vi "Read_HGB2.vi"(8 "error in (no error)":errorcluster, 11 "Task Array":refnum<k21>[](array[refnum])=["", ""]) -> (0 "error out":errorcluster={"status"=TRUE, "code"=-200478, "source"="Read_HGB.vi<append>\n<B>Task Name: </B>_unnamedTask<37>"}, 1 "NI 6001":waveform(dbl)[](array[waveform]), 3 "Data Main":waveform(dbl)[](array[waveform]))   [LabVIEW 2016]
uses:
  <vilib>/Utility/error.llb/DialogType.ctl
  <vilib>/DAQmx/read.llb/DAQmx Read (Analog 1D Wfm NChan NSamp).vi
  <vilib>/DAQmx/miscellaneous.llb/DAQmx Fill In Error Info.vi
panel:
  out "Accelerometer Data":waveform(dbl)[](array[waveform])
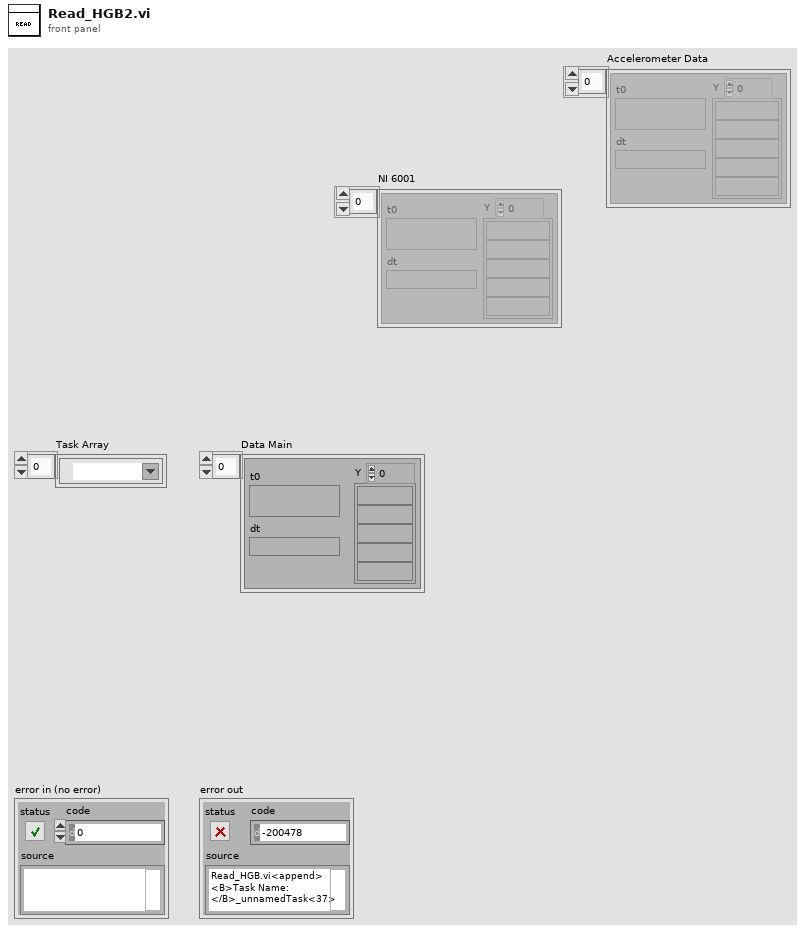
[diagram p1: front panel]
types:
  T1 = typedef "DialogType.ctl" = u16
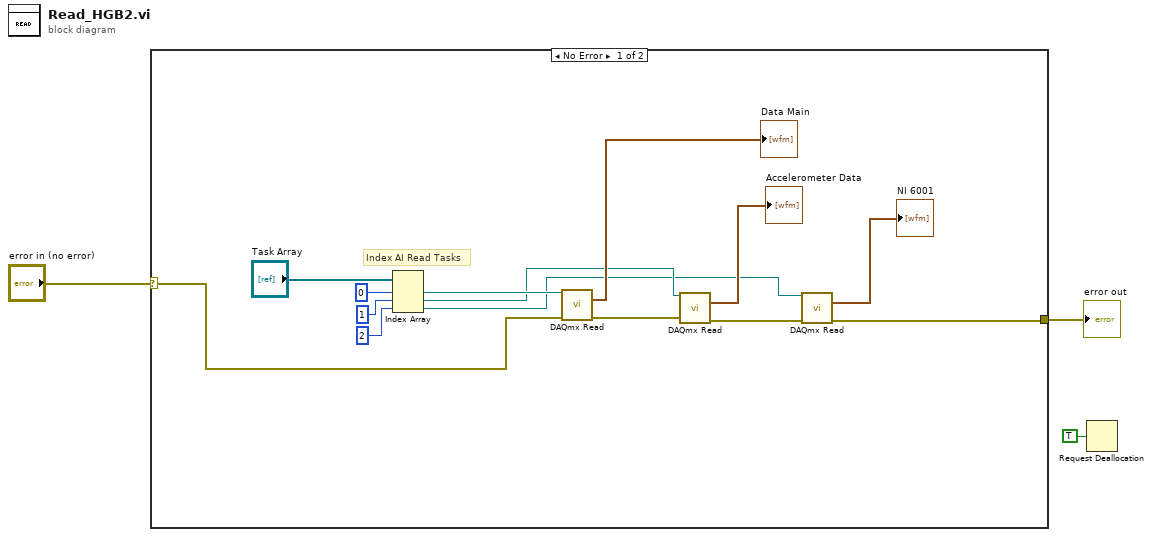
[diagram p0: block diagram]
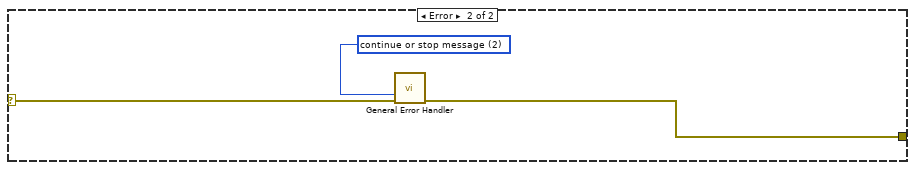
[diagram p2: hidden frame]
diagram:
  n1 = case shown="No Error" "error in (no error)" {
    selector: "error in (no error)" -> [w13 w19]
    tunnel: [w10 w18] -> w3
    frame No Error {
      # "Index AI Read Tasks"
      n2 = Index Array(array="Task Array", index #1=0 ("index"), index #2=1 ("index"), index #3=2 ("index")) -> (element #1=w17:refnum<k21>, element #2=w5:refnum<k21>, element #3=w4:refnum<k21>)
      n3 = call-poly <vilib>:"DAQmx Read.vi"("task/channels in"=w17, "error in"=w13) -> ("data"=→"Data Main":waveform(dbl)[], "error out"=w7:errorcluster)  [unwired: 11 in, 1 out]
      n4 = call-poly <vilib>:"DAQmx Read.vi"("task/channels in"=w5, "error in"=w7) -> ("data"=→"Accelerometer Data":waveform(dbl)[], "error out"=w6:errorcluster)  [unwired: 11 in, 1 out]
      n5 = call-poly <vilib>:"DAQmx Read.vi"("task/channels in"=w4, "error in"=w6) -> ("data"=→"NI 6001":waveform(dbl)[], "error out"=w10:errorcluster)  [unwired: 11 in, 1 out]
    }
    frame Error {
      w20 = T1 2 items=["no dialog", "OK message", "continue or stop message", "OK message + warnings", "continue/stop + warnings"] ("type of dialog (OK msg:1)")
      n6 = call <vilib>:"General Error Handler.vi"("type of dialog (OK msg:1)"=w20, "error in (no error)"=w19) -> ("error out"=w18:errorcluster)  [unwired: 9 in, 4 out]
    }
  }
  "error out" <- w3
  n7 = Request Deallocation(TRUE ("flag")) -> ()
